vi "BaudDetect-Make Success Info.vi"(10 "Normal":bool, 11 "list":refnum<vi>) -> (3 "Info":string)   [LabVIEW 2011]
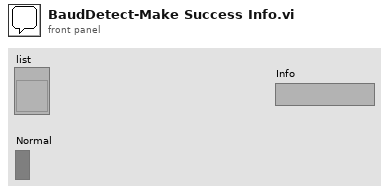
[diagram p1: front panel]
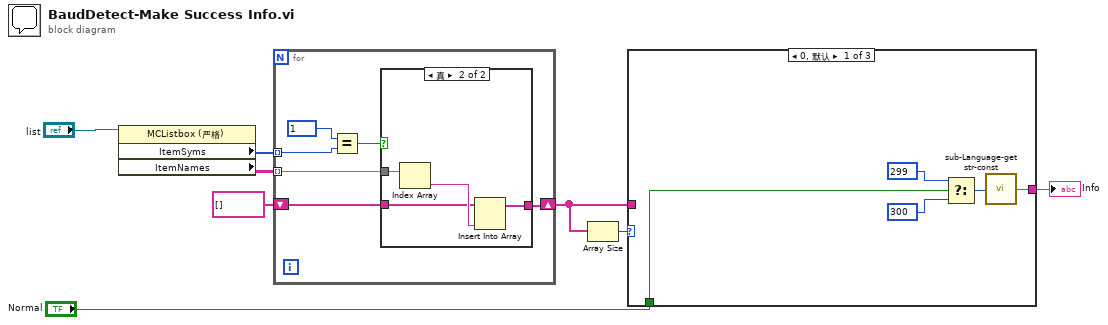
[diagram p0: block diagram]
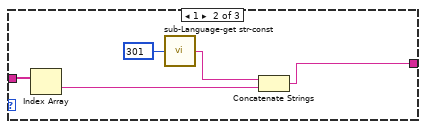
[diagram p2: hidden frame]
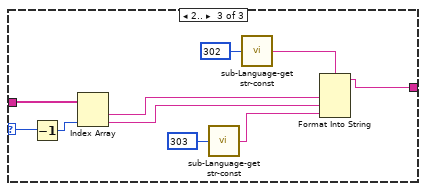
[diagram p3: hidden frame]
diagram:
  n1 = property class="MCListbox (严格)"(reference="list") -> ("ItemSyms"=w7:i32[], "ItemNames"=w6:string[][])  [unwired: 1 in, 2 out]
  n2 = for {
    tunnel: w7 -> [w14] mode=indexing
    tunnel: w6 -> [w11] mode=indexing
    shift-right: [w10] -> w3
    shift-left: string[] [] -> [w9]
    n3 = Equal?(x=1, y=w14) -> (x = y?=w12:bool)
    n4 = case shown="真" w12 {
      tunnel: w11 -> [_ w19]
      tunnel: [w15 w17] -> w10
      tunnel: w9 -> [w15 w16]
      frame False {
      }
      frame True {
        n5 = Index Array(array=w19) -> (element=w18:string)  [unwired: 1 in]
        n6 = Insert Into Array(array=w16, new element=w18) -> (w17:string[])  [unwired: 1 in]
      }
    }
  }
  n7 = Array Size(array=w3) -> (size(s)=w4:i32)
  n8 = case shown="0, 默认" w4 {
    selector: w4 -> [_ _ w38]
    tunnel: w3 -> [_ w29 w39]
    tunnel: "Normal" -> [w24 _ _]
    tunnel: [w22 w27 w34] -> w1
    frame 0, Default {
      n9 = Select(t=u32 299 ("sid"), s=w24, f=u32 300 ("sid")) -> (s? t:f=w23:u32)
      n10 = call "sub-Language-get str-const.vi"("sid"=w23) -> ("str"=w22:string)
    }
    frame 1 {
      n11 = Index Array(array=w29) -> (element=w28:string)  [unwired: 1 in]
      n12 = call "sub-Language-get str-const.vi"("sid"=u32 301) -> ("str"=w25:string)
      n13 = Concatenate Strings(w25, w28) -> (w27:string)
    }
    frame 2.. {
      n14 = Decrement(x=w38) -> (x-1=w37:i32)
      n15 = Index Array(array=w39, index #2=w37) -> (element #1=w36:string, element #2=w35:string)  [unwired: 1 in]
      n16 = call "sub-Language-get str-const.vi"("sid"=u32 303) -> ("str"=w30:string)
      n17 = call "sub-Language-get str-const.vi"("sid"=u32 302) -> ("str"=w32:string)
      n18 = Format Into String(format string=w32, w36, w35, w30) -> (resulting string=w34:string)  [unwired: 2 in, 1 out]
    }
  }
  "Info" <- w1
